vi "Autonomous Independent.vi"() -> ()   [LabVIEW 2017]
doc: "This VI is called when autonomous begins, and will automatically be terminated when autonomous ends. You can carry out timed or sensor driven robot movement independently without needing to return to the caller."
uses:
  <vilib>/Rock Robotics/Network Tables/NT Read String.vi
  Auto/AutoGlobals.vi
panel:
  in  "XCoordinates":dbl[](array[numeric])
  in  "YCoordinates":dbl[](array[numeric])
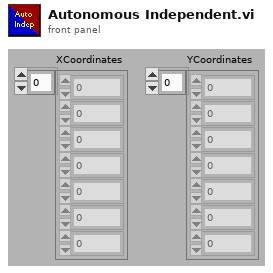
[diagram p1: front panel]
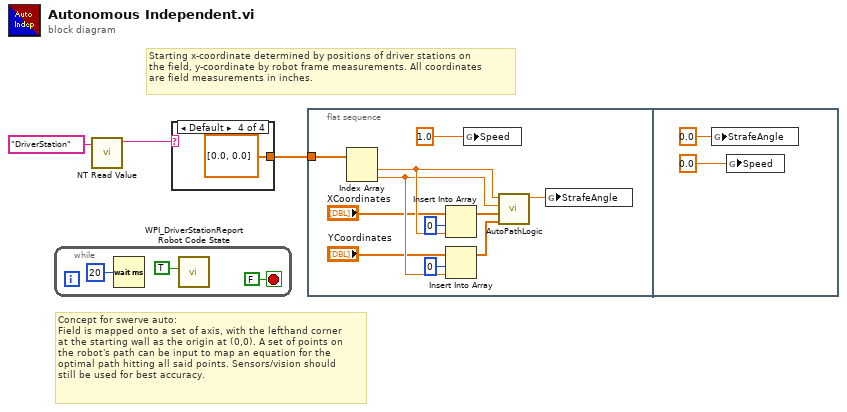
[diagram p0: block diagram]
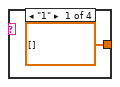
[diagram p2: hidden frame]
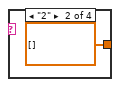
[diagram p3: hidden frame]
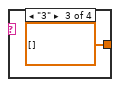
[diagram p4: hidden frame]
diagram:
  # "Starting x-coordinate determined by positions of driver stations on\nthe field, y-coordinate by robot frame measurements. All coordinates\nare field measurements in inches."
  # "Concept for swerve auto:\nField is mapped onto a set of axis, with the lefthand corner\nat the starting wall as the origin at (0,0). A set of points on\nthe robot's path can be input to map an equation for the\noptimal path hitting all said points. Sensors/vision should\nstill be used for best accuracy."
  n1 = while {
    stop <- FALSE stop-if-true
    n2 = Wait (ms)(milliseconds to wait=u32 20) -> ()  [unwired: 1 out]
    n3 = call <vilib>:"WPI_DriverStationReport Robot Code State.vi"("Autonomous"=TRUE) -> ()  [unwired: 10 in, 1 out]
  }
  n4 = call-poly <vilib>:"NT Read Value.vi"("Name"="DriverStation") -> ("String"=w2:string)  [unwired: 9 in, 1 out]
  n5 = case shown="Default" w2 {
    tunnel: [dbl[] [] dbl[] [] dbl[] [] dbl[] [0.0, 0.0]] -> w1
    frame "1" {
    }
    frame "2" {
    }
    frame "3" {
    }
    frame Default {
    }
  }
  n6 = flat-sequence {
    tunnel: w1 -> [w19]
    frame #0 {
      n7 = Index Array(array=w19) -> (element #1=w14:dbl, element #2=w13:dbl)  [unwired: 2 in]
      n8 = Insert Into Array(array="XCoordinates", index=0, new element=w14) -> (w17:dbl[])
      n9 = Insert Into Array(array="YCoordinates", index=0, new element=w13) -> (w15:dbl[])
      n10 = global write "AutoGlobals.vi" "Speed"(1.0 ("SwerveSpeeds")) -> ()
      n11 = call "AutoPathLogic.vi"("YCoordinates"=w15, "XCoordinates"=w17, "Y"=w13, "X"=w14) -> ("Angle"=w21:dbl)  [unwired: 7 in]
      n12 = global write "AutoGlobals.vi" "StrafeAngle"(w21) -> ()
    }
    frame #1 {
      n13 = global write "AutoGlobals.vi" "StrafeAngle"(0.0 ("SwerveAngles")) -> ()
      n14 = global write "AutoGlobals.vi" "Speed"(0.0 ("SwerveSpeeds")) -> ()
    }
  }
